vi "Tracking Chart Refresh.vi"(4 "Data":string[](array[string]), 5 "N Items":u8, 6 "Signal Names":string[](array[string]), 7 "_Table":refnum<vi>, 8 "Signal Units":string[](array[string]), 9 "Slider Min":sgl[](array[numeric]), 10 "Slider Max":sgl[](array[numeric])) -> (1 "Short Signal Names":string[](array[string]))   [LabVIEW 2015, in "ECS-Host.lvlib"]
uses:
  ECS-Host.lvlib
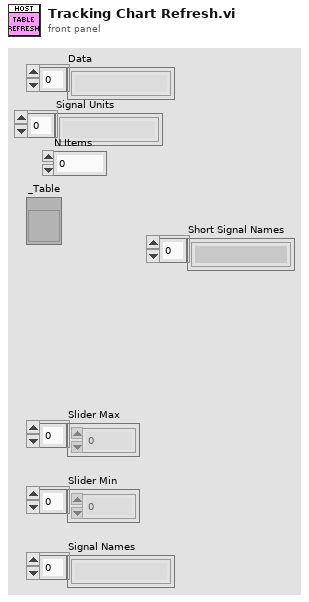
[diagram p1: front panel]
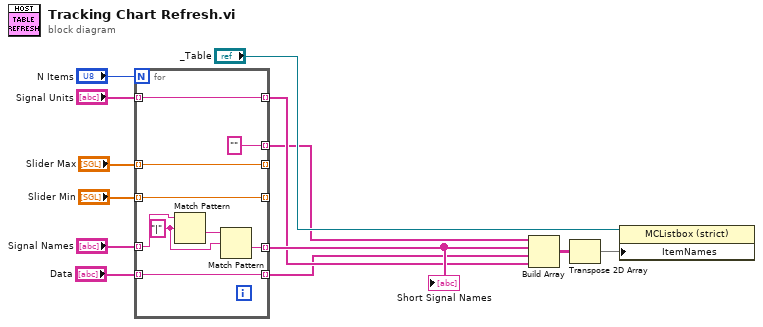
[diagram p0: block diagram]
diagram:
  n1 = for {
    N: "N Items" -> [_]
    tunnel: "Slider Max" -> [w22] mode=indexing
    tunnel: "Slider Min" -> [w21] mode=indexing
    tunnel: [w19] -> w10 mode=indexing
    tunnel: [w22] -> _ mode=indexing
    tunnel: [w21] -> _ mode=indexing
    tunnel: [w16] -> w13 mode=indexing
    tunnel: "Signal Names" -> [w15] mode=indexing
    tunnel: [w20] -> w9 mode=indexing
    tunnel: "Data" -> [w20] mode=indexing
    tunnel: "Signal Units" -> [w19] mode=indexing
    tunnel: ["" ("delimiter (Tab)")] -> w3 mode=indexing
    w18 = "|" ("regular expression")
    n2 = Match Pattern(string=w15, regular expression=w18) -> (after substring=w17:string)  [unwired: 1 in, 3 out]
    n3 = Match Pattern(string=w17, regular expression=w18) -> (after substring=w16:string)  [unwired: 1 in, 3 out]
  }
  "Short Signal Names" <- w13
  n4 = Build Array(w3, w13, w9, w10) -> (w11:string[][])
  n5 = Transpose 2D Array(2D array=w11) -> (transposed array=w12:string[][])
  n6 = property on="Property Node" class="MCListbox (strict)"(reference="_Table", "ItemNames"=w12) -> ()  [unwired: 1 in, 2 out]
